vi "UHR-Fleezers Control (host) - 10.4.vi"() -> ()   [LabVIEW 2011] (continued)
                    n400 = Compound Arithmetic op=OR(w626, w627, w625) -> (w624:bool)
                    n401 = Select(t=FALSE, s=w623, f=w624) -> (s? t:f=w621:bool)
                    n402 = Not(x=w617) -> (.not. x?=w616:bool)
                    n403 = node-c288() -> ()  [unwired: 1 in, 1 out]
                    n404 = And(x=w620, y=w616) -> (x .and. y?=w618:bool)
                    n405 = Or(x=w621, y=w617) -> (x .or. y?=w619:bool)
                  }
                  n406 = node-c288(w611) -> ()  [unwired: 1 out]
                }
                frame #3 {
                  n407 = case shown="True" w636 {
                    tunnel: w635 -> [_ w638]
                    tunnel: w634 -> [_ w637]
                    frame False {
                    }
                    frame True {
                      n408 = flat-sequence {
                        tunnel: w638 -> [w641]
                        tunnel: w637 -> [w640]
                        frame #0 {
                          n409 = local read "Saved Stage Positions"() -> (w644:dbl[][])
                          n410 = local write "Cancel dwell"(FALSE ("Cancel dwell")) -> ()
                          n411 = call "move to saved stage position.vi"("error in"=w640, "Stage VISA resource name in"=w641, "Position"="Return Stage \nPosition", "Saved Stage Positions"=w644) -> ("error out"=w642:errorcluster)  [unwired: 1 out]
                          n412 = local write "Stage Control Serial Error"(w642) -> ()
                        }
                        frame #1 {
                          n413 = case shown="True" "Green ON \nafter return?" {
                            frame False {
                            }
                            frame True {
                              n414 = property on="Green Laser ON/Interlacing" class="Bool (strict)"("Val(Sgnl)"=TRUE ("Value (Signaling)")) -> ()  [unwired: 2 in, 2 out]
                            }
                          }
                          n415 = case shown="True" "Move trap \nafter return move?" {
                            frame False {
                            }
                            frame True {
                              n416 = property on="Trap Delta (MHz)" class="DigNum (strict)"("Val(Sgnl)"="Dip Trap Delta 2 (MHz)") -> ()  [unwired: 2 in, 2 out]
                            }
                          }
                          n417 = property on="Sample Channel\nFlow" class="Bool (strict)"("Val(Sgnl)"="Flow ON\nafter dip?") -> ()  [unwired: 2 in, 2 out]
                          n418 = case shown="True" "Save data\nafter return move?" {
                            frame False {
                            }
                            frame True {
                              n419 = property on="Start Saving" class="Bool (strict)"("Val(Sgnl)"=TRUE ("Value (Signaling)")) -> ()  [unwired: 2 in, 2 out]
                            }
                          }
                        }
                        frame #2 {
                          n420 = node-c288() -> (w653:T21)  [unwired: 4 in]
                          n421 = timed-loop {
                            timing: w653 -> [_]
                            timing-out: [_] -> w652
                            i -> [w665]
                            stop <- w655 stop-if-true
                            n422 = node-c288() -> ()  [unwired: 1 in, 1 out]
                            n423 = local read "Dump Beads"() -> (w654:bool)
                            n424 = Greater Or Equal?(x=w665, y="Dwell Duration (s)") -> (x >= y?=w660:bool)
                            n425 = local read "Dip for Protein"() -> (w657:bool)
                            n426 = Not(x=w657) -> (.not. x?=w656:bool)
                            n427 = Compound Arithmetic op=OR(w660, "Cancel dwell", w656) -> (w659:bool)
                            n428 = node-c288() -> ()  [unwired: 1 in, 1 out]
                            n429 = Select(t=FALSE, s="Pause dwell \ntimer", f=w659) -> (s? t:f=w662:bool)
                            n430 = Or(x=w662, y=w654) -> (x .or. y?=w655:bool)
                          }
                          n431 = node-c288(w652) -> ()  [unwired: 1 out]
                        }
                      }
                    }
                  }
                }
                frame #4 {
                  n432 = local read "Dip for Protein"() -> (w673:bool)
                  n433 = local read "Dump Beads"() -> (w670:bool)
                  n434 = local write "Cancel dwell"(FALSE ("Cancel dwell")) -> ()
                  n435 = Not(x=w673) -> (.not. x?=w674:bool)
                  n436 = Not(x="Cont. Repeat Dipping?") -> (.not. x?=w676:bool)
                  n437 = Compound Arithmetic op=OR(w674, w676, w670) -> (w672:bool)
                }
              }
            }
          }
        }
      }
      event "Profile": Value Change {
        n438 = event-data() -> ()  [unwired: 1 in, 5 out]
        n439 = flat-sequence {
          tunnel: w685 -> [w688]
          tunnel: w684 -> [w696]
          tunnel: [w690] -> w683
          tunnel: [w689] -> w682
          tunnel: [w687] -> w680
          tunnel: [w686] -> w677
          tunnel: w683 -> [w703]
          tunnel: w682 -> [w702]
          tunnel: [w700] -> w681
          tunnel: w680 -> [w701]
          tunnel: [w699] -> w679
          tunnel: [w698] -> w678
          tunnel: w677 -> [w698]
          tunnel: w681 -> [w707]
          tunnel: w679 -> [w706]
          tunnel: w678 -> [w705]
          frame #0 {
            n440 = call "Read Stage Position.vi"("error in"=w696, "VISA resource name in"=w688) -> ("Current Position"=w686:cluster{dbl, dbl, dbl}, "error out"=w689:errorcluster, "VISA resource name out"=w687:refnum<visa-resource-name>)  [unwired: 1 out]
            "Current Position" <- w686
            n441 = local write "Stage Control Serial Error"(w689) -> ()
            n442 = Unbundle(w686) -> (w693:dbl, w695:dbl, w691:dbl)
            n443 = Add(x=w695, y="Y change (mm)") -> (x+y=w692:dbl)
            n444 = Bundle(w693, w692, w691) -> (w690:cluster{dbl, dbl, dbl})  [unwired: 1 in]
          }
          frame #1 {
            # "move to new position and start saving"
            n445 = local write "Stage Moving"(TRUE ("Stage Moving")) -> ()
            n446 = local write "Start Saving"(TRUE ("Start Saving")) -> ()
            n447 = call "Set Stage Position.vi"("Position"=w703, "error in"=w702, "VISA resource name in"=w701) -> ("error out"=w699:errorcluster, "VISA resource name out"=w700:refnum<visa-resource-name>)  [unwired: 1 out]
          }
          frame #2 {
            # "go back to start"
            n448 = call "Set Stage Position.vi"("Position"=w705, "error in"=w706, "VISA resource name in"=w707) -> ()  [unwired: 3 out]
          }
          frame #3 {
            # "stop saving"
            n449 = local write "Stop Saving"(TRUE ("Stop Saving")) -> ()
            n450 = local write "Stage Moving"(FALSE ("Stage Moving")) -> ()
          }
        }
      }
      event "Move to Position 1", "Move to Position 2", "Move to Position 3", "Move to Position 4", "Move to Position 5", "Lower Ch. Cap.": Value Change {
        n451 = event-data() -> ()  [unwired: 1 in, 5 out]
        n452 = Or(x="Move to Position 5", y="Lower Ch. Cap.") -> (x .or. y?=w713:bool)
        n453 = Build Array("Move to Position 1", "Move to Position 2", "Move to Position 3", "Move to Position 4", w713) -> (w716:bool[])
        n454 = Boolean Array To Number(Boolean array=w716) -> (number=w715:u32)
        n455 = Logarithm Base 2(1:w715) -> (0:w714:dbl)
        n456 = flat-sequence {
          tunnel: w714 -> [w725]
          tunnel: w711 -> [w723]
          tunnel: w710 -> [w722]
          frame #0 {
            n457 = local read "Saved Stage Positions"() -> (w733:dbl[][])
            n458 = Array Subset(array=w733, index (row)=w725, length (row)=1 ("length"), index (col)=1 ("index"), length (col)=3 ("length")) -> (w730:dbl[][])
            n459 = Reshape Array(w730, 3 ("dimension size")) -> (w728:dbl[])
            n460 = Array To Cluster(array=w728) -> (cluster=w727:cluster{"[0]":dbl, "[1]":dbl, "[2]":dbl})
            n461 = call "Set Stage Position.vi"("Position"=w727, "error in"=w722, "VISA resource name in"=w723) -> ("error out"=w726:errorcluster)  [unwired: 2 out]
            n462 = local write "Stage Moving"(TRUE ("Stage Moving")) -> ()
            n463 = local write "Stage Control Serial Error"(w726) -> ()
          }
          frame #1 {
            n464 = local write "Stage Moving"(FALSE ("Stage Moving")) -> ()
            n465 = call <vilib>:"Beep.vi"() -> ()  [unwired: 3 in, 9 out]
          }
        }
      }
      event "Got ADig bead": Value Change {
        n466 = event-data() -> ()  [unwired: 1 in, 5 out]
        n467 = local read "Cap 1 Samp Flow ON"() -> (w736:bool)
        n468 = flat-sequence {
          tunnel: w736 -> [w738]
          frame #0 {
            n469 = case shown="True" w738 {
              frame False {
              }
              frame True {
                n470 = property on="Sample Channel\nFlow" class="Bool (strict)"("Val(Sgnl)"=TRUE ("Value (Signaling)")) -> ()  [unwired: 2 in, 2 out]
              }
            }
          }
          frame #1 {
            n471 = property on="Move Cap. 1 (DNA Bottom)" class="Bool (strict)"("Val(Sgnl)"=TRUE ("Value (Signaling)")) -> ()  [unwired: 2 in, 2 out]
            n472 = property on="Inject Pump 3" class="Bool (strict)"("Val(Sgnl)"=FALSE ("Value (Signaling)")) -> ()  [unwired: 2 in, 2 out]
          }
        }
      }
      event "Take Force FB Data\nScript": Value Change {
        n473 = event-data() -> ()  [unwired: 1 in, 5 out]
        n474 = flat-sequence {
          tunnel: w747 -> [w751]
          tunnel: w748 -> [w752]
          tunnel: [w752] -> w743
          tunnel: [w751] -> w742
          tunnel: w743 -> [w755]
          tunnel: w742 -> [w754]
          tunnel: ["Trap Trig Fl."] -> w744
          tunnel: [w780] -> w745
          tunnel: w744 -> [w780]
          tunnel: [w783] -> w746
          tunnel: w745 -> [w783]
          tunnel: w746 -> [w786]
          frame #0 {
            n475 = property on="Trap Delta (MHz)" class="DigNum (strict)"("Val(Sgnl)"="Trap Delta Before Moving") -> ()  [unwired: 2 in, 2 out]
          }
          frame #1 {
            n476 = local read "Saved Stage Positions"() -> (w757:dbl[][])
            n477 = local write "FB Trap Pos Offset"(0.0 ("FB Trap Pos Offset")) -> ()
            n478 = property on="Trap Pos. FB Offset Factor" class="DigNum (strict)"("Val(Sgnl)"=i64 0 ("Value (Signaling)")) -> ()  [unwired: 2 in, 2 out]
            n479 = local write "Stage Moving"(TRUE ("Stage Moving")) -> ()
            n480 = call "move to saved stage position.vi"("error in"=w754, "Stage VISA resource name in"=w755, "Position"="Stage Position To Establish FB", "Saved Stage Positions"=w757) -> ("error out"=w753:errorcluster)  [unwired: 1 out]
            n481 = local write "Stage Control Serial Error"(w753) -> ()
          }
          frame #2 {
            n482 = call <vilib>:"Beep.vi"() -> ()  [unwired: 3 in, 9 out]
            n483 = Multiply(x="Wait (s)", y=u32 1000 ("milliseconds to wait")) -> (x*y=w763:u32)
            n484 = property on="Trap Delta (MHz)" class="DigNum (strict)"("Val(Sgnl)"="Starting \nTrap Delta (MHz)") -> ()  [unwired: 2 in, 2 out]
            n485 = local write "Stage Moving"(FALSE ("Stage Moving")) -> ()
            n486 = Wait (ms)(milliseconds to wait=w763) -> ()  [unwired: 1 out]
            n487 = property on="Tab Control 2" class="TabCtl (strict)"("Val(Sgnl)"=T6."Feedback on Trap Position" ("Value (Signaling)")) -> ()  [unwired: 2 in, 2 out]
            n488 = property on="Tab Control" class="TabCtl (strict)"("Val(Sgnl)"=T4."Trap Control (RF)" ("Value (Signaling)")) -> ()  [unwired: 2 in, 2 out]
          }
          frame #3 {
            n489 = property on="Set Reading to\nSetpoint" class="Bool (strict)"("Val(Sgnl)"=TRUE ("Value (Signaling)")) -> ()  [unwired: 2 in, 2 out]
            n490 = Wait (ms)(milliseconds to wait=u32 500) -> ()  [unwired: 1 out]
          }
          frame #4 {
            n491 = property on="Trap Pos. FB ON" class="Bool (strict)"("Val(Sgnl)"=TRUE ("Value (Signaling)")) -> ()  [unwired: 2 in, 2 out]
            n492 = Wait (ms)(milliseconds to wait=u32 250) -> ()  [unwired: 1 out]
          }
          frame #5 {
            n493 = case shown="False" "Trap Trig Fl." {
              frame False {
                n494 = case shown="True" "Green ON after FB ON?" {
                  selector: "Green ON after FB ON?" -> [_ w779]
                  frame False {
                  }
                  frame True {
                    n495 = property on="Green Laser ON/Interlacing" class="Bool (strict)"("Val(Sgnl)"=w779) -> ()  [unwired: 2 in, 2 out]
                  }
                }
              }
              frame True {
              }
            }
            n496 = case shown="False" "Remove Action Offset" {
              tunnel: TRUE ("Value (Signaling)") -> [w776 w777]
              frame False {
                n497 = property on="Remove Unwinding Offset" class="Bool (strict)"("Val(Sgnl)"=w776) -> ()  [unwired: 2 in, 2 out]
              }
              frame True {
                n498 = property on="Remove Action Offset" class="Bool (strict)"("Val(Sgnl)"=w777) -> ()  [unwired: 2 in, 2 out]
              }
            }
            n499 = Wait (ms)(milliseconds to wait=u32 250) -> ()  [unwired: 1 out]
          }
          frame #6 {
            n500 = property on="Start Saving" class="Bool (strict)"("Val(Sgnl)"=TRUE ("Value (Signaling)")) -> ()  [unwired: 2 in, 2 out]
            n501 = Wait (ms)(milliseconds to wait=u32 5000) -> ()  [unwired: 1 out]
          }
          frame #7 {
            n502 = property on="Rem fb disp offset" class="Bool (strict)"("Val(Sgnl)"=TRUE ("Value (Signaling)")) -> ()  [unwired: 2 in, 2 out]
            n503 = Wait (ms)(milliseconds to wait=u32 100) -> ()  [unwired: 1 out]
          }
          frame #8 {
            n504 = case shown="True" w786 {
              frame False {
              }
              frame True {
                n505 = local write "Trap Trig. Fl."(TRUE ("Value (Signaling)")) -> ()
              }
            }
          }
          frame #9 {
            n506 = case shown="True" "Start dipping after?" {
              frame False {
              }
              frame True {
                n507 = property on="Dip for Protein" class="Bool (strict)"("Val(Sgnl)"=TRUE ("Value (Signaling)")) -> ()  [unwired: 2 in, 2 out]
                n508 = local write "Scripts"(T1."Dipping" ("Scripts")) -> ()
              }
            }
          }
        }
      }
      event "Test move stage": Value Change {
        n509 = event-data() -> ()  [unwired: 1 in, 5 out]
        n510 = local read "Saved Stage Positions"() -> (w791:dbl[][])
        n511 = call "move to saved stage position.vi"("error in"=w792, "Stage VISA resource name in"=w793, "Saved Stage Positions"=w791) -> ()  [unwired: 1 in, 2 out]
      }
      event "Got DNA bead": Value Change {
        n512 = event-data() -> ()  [unwired: 1 in, 5 out]
        n513 = flat-sequence {
          frame #0 {
            n514 = local read "Daq spot flow on"() -> (w796:bool)
            n515 = case shown="True" w796 {
              frame False {
              }
              frame True {
                n516 = property on="Sample Channel\nFlow" class="Bool (strict)"("Val(Sgnl)"=TRUE ("Value (Signaling)")) -> ()  [unwired: 2 in, 2 out]
              }
            }
          }
          frame #1 {
            n517 = property on="Cal/Data Acq. Spot" class="Bool (strict)"("Val(Sgnl)"=TRUE ("Value (Signaling)")) -> ()  [unwired: 2 in, 2 out]
            n518 = property on="Inject Pump 1" class="Bool (strict)"("Val(Sgnl)"=FALSE ("Value (Signaling)")) -> ()  [unwired: 2 in, 2 out]
          }
        }
      }
      event "Take Stepping Data": Value Change {
        n519 = event-data() -> ()  [unwired: 1 in, 5 out]
        n520 = local read "Save ave N"() -> (w808:dbl)
        n521 = flat-sequence {
          tunnel: w808 -> [w810]
          tunnel: [w810] -> w803
          tunnel: [w812] -> w804
          tunnel: w803 -> [w812]
          tunnel: [w814] -> w805
          tunnel: w804 -> [w814]
          tunnel: [w817] -> w806
          tunnel: w805 -> [w817]
          tunnel: [w819] -> w807
          tunnel: w806 -> [w819]
          tunnel: [w821] -> w801
          tunnel: w807 -> [w821]
          tunnel: w801 -> [w824]
          tunnel: [w824] -> w800
          tunnel: w800 -> [w825]
          tunnel: [w825] -> w802
          tunnel: w802 -> [w831]
          frame #0 {
            n522 = property on="Save ave N" class="DigNum (strict)"("Val(Sgnl)"="Save ave factor") -> ()  [unwired: 2 in, 2 out]
          }
          frame #1 {
            n523 = Wait (ms)(milliseconds to wait=u32 100) -> ()  [unwired: 1 out]
          }
          frame #2 {
            n524 = local read "Offset 2 Start (MHz)"() -> (w816:dbl)
            n525 = property on="Saved AOD Raster Scan Parameter Sets" class="Arr (strict)"("Index Values"=u32[] [2]) -> ()  [unwired: 2 in, 2 out]
            n526 = property on="Trap Delta (MHz)" class="DigNum (strict)"("Val(Sgnl)"=w816) -> ()  [unwired: 2 in, 2 out]
          }
          frame #3 {
            n527 = property on="Load parameters" class="Bool (strict)"("Val(Sgnl)"=TRUE ("Value (Signaling)")) -> ()  [unwired: 2 in, 2 out]
          }
          frame #4 {
            n528 = Wait (ms)(milliseconds to wait=u32 100) -> ()  [unwired: 1 out]
          }
          frame #5 {
            n529 = property on="Trap Raster Scan" class="Bool (strict)"("Val(Sgnl)"=TRUE ("Value (Signaling)")) -> ()  [unwired: 2 in, 2 out]
          }
          frame #6 {
            n530 = Wait (ms)(milliseconds to wait=u32 1000) -> ()  [unwired: 1 out]
          }
          frame #7 {
            n531 = while {
              stop <- w828 stop-if-true
              n532 = local read "Raster Scanning..."() -> (w830:bool)
              n533 = local read "Saving..."() -> (w829:bool)
              n534 = Not(x=w829) -> (.not. x?=w826:bool)
              n535 = Not(x=w830) -> (.not. x?=w827:bool)
              n536 = And(x=w827, y=w826) -> (x .and. y?=w828:bool)
            }
          }
          frame #8 {
            n537 = property on="Save ave N" class="DigNum (strict)"("Val(Sgnl)"=w831) -> ()  [unwired: 2 in, 2 out]
          }
        }
      }
      event "Step Size (nm)": Value Change {
        n538 = event-data() -> ()  [unwired: 1 in, 5 out]
        n539 = flat-sequence {
          frame #0 {
            n540 = property on="Saved AOD Raster Scan Parameter Sets" class="Arr (strict)"("Index Values"=u32[] [1]) -> ()  [unwired: 2 in, 2 out]
          }
          frame #1 {
            n541 = Multiply(x="N Steps", y="Step Size (nm)") -> (x*y=w833:dbl)
            n542 = property on="Scan Speed AOD (nm/s) 2" class="DigNum (strict)"("Value"="Step Size (nm)") -> ()  [unwired: 2 in, 2 out]
            n543 = property on="Step Size AOD (nm) 2" class="DigNum (strict)"("Value"="Step Size (nm)") -> ()  [unwired: 2 in, 2 out]
            n544 = property on="Scan Range AOD (nm) 2" class="DigNum (strict)"("Value"=w833) -> ()  [unwired: 2 in, 2 out]
          }
        }
      }
      event "Take Detection Laser\nImage": Value Change {
        n545 = event-data() -> ()  [unwired: 1 in, 5 out]
        n546 = flat-sequence {
          tunnel: [w861] -> w851
          tunnel: [w860] -> w844
          tunnel: [w859] -> w836
          tunnel: [w864] -> w852
          tunnel: w851 -> [w864]
          tunnel: [w863] -> w845
          tunnel: w844 -> [w863]
          tunnel: [w862] -> w837
          tunnel: w836 -> [w862]
          tunnel: [w868] -> w853
          tunnel: w852 -> [w868]
          tunnel: [w867] -> w846
          tunnel: w845 -> [w867]
          tunnel: [w866] -> w838
          tunnel: w837 -> [w866]
          tunnel: [w874] -> w854
          tunnel: w853 -> [w874]
          tunnel: [w873] -> w847
          tunnel: w846 -> [w873]
          tunnel: [w872] -> w839
          tunnel: w838 -> [w872]
          tunnel: [w878] -> w855
          tunnel: w854 -> [w878]
          tunnel: [w877] -> w848
          tunnel: w847 -> [w877]
          tunnel: [w876] -> w840
          tunnel: w839 -> [w876]
          tunnel: [w882] -> w856
          tunnel: w855 -> [w882]
          tunnel: [w881] -> w849
          tunnel: w848 -> [w881]
          tunnel: [w880] -> w841
          tunnel: w840 -> [w880]
          tunnel: [w886] -> w857
          tunnel: w856 -> [w886]
          tunnel: [w885] -> w850
          tunnel: w849 -> [w885]
          tunnel: [w884] -> w842
          tunnel: w841 -> [w884]
          tunnel: w857 -> [w892]
          tunnel: w850 -> [w891]
          tunnel: [w889] -> w843
          tunnel: w842 -> [w889]
          tunnel: w843 -> [w893]
          frame #0 {
            n547 = local read "Green Laser ON/Interlacing"() -> (w861:bool)
            n548 = local read "Green laser mode"() -> (w860:enum32{"Laser ON", "Laser OFF", "Interlace"})
            n549 = local read "Green FB On/Off"() -> (w859:bool)
          }
          frame #1 {
            n550 = property on="Green FB On/Off" class="Bool (strict)"("Val(Sgnl)"=FALSE ("Value (Signaling)")) -> ()  [unwired: 2 in, 2 out]
          }
          frame #2 {
            n551 = property on="Green Laser ON/Interlacing" class="Bool (strict)"("Val(Sgnl)"=TRUE ("Value (Signaling)")) -> ()  [unwired: 2 in, 2 out]
            n552 = property on="Flip Green Filter" class="Bool (strict)"("Val(Sgnl)"=TRUE ("Value (Signaling)")) -> ()  [unwired: 2 in, 2 out]
            n553 = property on="Green laser mode" class="RadioBtnsControl (strict)"("Val(Sgnl)"=enum32{"Laser ON", "Laser OFF", "Interlace"}."Laser ON" ("Value (Signaling)")) -> ()  [unwired: 2 in, 2 out]
          }
          frame #3 {
            n554 = Wait (ms)(milliseconds to wait=u32 500) -> ()  [unwired: 1 out]
          }
          frame #4 {
            n555 = property on="Confocal Image" class="Bool (strict)"("Val(Sgnl)"=TRUE ("Value (Signaling)")) -> ()  [unwired: 2 in, 2 out]
          }
          frame #5 {
            n556 = Wait (ms)(milliseconds to wait=u32 2000) -> ()  [unwired: 1 out]
          }
          frame #6 {
            n557 = while {
              stop <- w887 stop-if-true
              n558 = local read "Saving..."() -> (w888:bool)
              n559 = Not(x=w888) -> (.not. x?=w887:bool)
            }
          }
          frame #7 {
            n560 = property on="Flip Green Filter" class="Bool (strict)"("Val(Sgnl)"=TRUE ("Value (Signaling)")) -> ()  [unwired: 2 in, 2 out]
            n561 = property on="Green Laser ON/Interlacing" class="Bool (strict)"("Val(Sgnl)"=w892) -> ()  [unwired: 2 in, 2 out]
            n562 = property on="Green laser mode" class="RadioBtnsControl (strict)"("Val(Sgnl)"=w891) -> ()  [unwired: 2 in, 2 out]
          }
          frame #8 {
            n563 = property on="Green FB On/Off" class="Bool (strict)"("Val(Sgnl)"=w893) -> ()  [unwired: 2 in, 2 out]
          }
        }
      }
      event "Stop All": Value Change {
        n564 = event-data() -> ()  [unwired: 1 in, 5 out]
        n565 = local read "Stop All"() -> (w894:bool)
      }
    }
    n566 = node-c288() -> ()  [unwired: 1 in, 1 out]
  }
  n567 = node-c288(2 ("Processor")) -> (w80:T21)  [unwired: 3 out]
  n568 = timed-loop "Control parameters (event loop)" {
    tunnel: w38 -> [w899]
    shift-right: [w898] -> _
    shift-left: errorcluster {"status"=FALSE, "code"=0, "source"=""} ("error out") -> [w897]
    tunnel: [w896] -> _
    timing: w80 -> [_]
    timing-out: [_] -> w79
    tunnel: w52 -> [w895]
    stop <- w896 stop-if-true
    n569 = node-c288() -> ()  [unwired: 2 out]
    n570 = event shown="[54] \"11\": Value Change" {
      selector: _ -> [_ _ _ _ _ _ _ _ _ _ _ _ _ _ _ _ _ _ _ _ _ _ _ _ _ _ _ _ _ _ _ _ _ _ _ _ _ _ _ _ _ _ _ _ _ _ _ _ _ _ _ _ _ _ _ _ _ _ _ _ _ _ _]
      dyn-events: _ -> [_ _ _ _ _ _ _ _ _ _ _ _ _ _ _ _ _ _ _ _ _ _ _ _ _ _ _ _ _ _ _ _ _ _ _ _ _ _ _ _ _ _ _ _ _ _ _ _ _ _ _ _ _ _ _ _ _ _ _ _ _ _ _]
      timeout: _ -> [_ _ _ _ _ _ _ _ _ _ _ _ _ _ _ _ _ _ _ _ _ _ _ _ _ _ _ _ _ _ _ _ _ _ _ _ _ _ _ _ _ _ _ _ _ _ _ _ _ _ _ _ _ _ _ _ _ _ _ _ _ _ _]
      tunnel: w899 -> [w937 _ _ _ w974 _ w996 _ _ _ _ w1062 _ _ w1105 w1111 w1116 w1122 w1158 w1176 w1183 w1194 w1198 w1209 w1220 w1231 w1242 w1253 w1264 w1291 w1385 w1392 w1430 _ w1465 w1469 w1480 w1484 w1488 _ w1496 _ _ _ _ _ _ _ w1667 _ w1684 _ w1691 w1709 _ w1716 w1724 w1739 w1748 w1751 w1756 _ w1772]
      tunnel: [w936 _ _ _ w964 _ w995 _ _ w1027 _ w1041 _ _ w1104 w1107 w1113 w1119 w1157 w1174 w1182 w1192 _ w1203 w1214 w1225 w1236 w1247 w1258 w1289 w1383 w1390 w1428 _ w1463 w1467 w1470 w1482 w1486 _ w1494 _ _ _ _ _ _ _ w1665 _ _ _ _ w1706 _ _ _ _ _ _ _ _ _] -> w898
      tunnel: w897 -> [w935 _ _ _ w973 _ w994 _ _ w1027 _ w1061 _ _ w1103 w1106 w1112 w1118 w1156 w1175 w1181 w1193 w1197 w1208 w1219 w1230 w1241 w1252 w1263 w1290 w1384 w1391 w1429 _ w1464 w1468 w1479 w1483 w1487 _ w1495 _ _ _ _ _ _ _ w1666 _ w1683 _ w1690 w1708 _ w1715 w1723 w1738 w1747 w1750 w1755 _ w1771]
      tunnel: [_ _ _ _ _ _ _ _ _ w1026 _ _ _ _ _ _ _ _ _ _ _ _ _ _ _ _ _ _ _ _ _ _ _ _ _ _ _ _ _ _ _ _ _ _ _ _ _ _ _ _ _ _ _ _ _ _ _ _ _ _ _ _ _] -> w896
      tunnel: [_ _ _ _ _ _ _ "Round T1 X" _ _ _ _ _ _ _ _ _ _ _ _ _ _ _ _ _ _ _ _ _ _ _ _ _ _ _ _ _ _ _ _ _ _ _ _ _ _ _ _ _ _ _ _ _ _ _ _ _ _ _ _ _ _ _] -> _
      tunnel: [_ _ _ "Adjust Scale\nto Mean" _ _ _ _ _ _ _ _ _ _ _ _ _ _ _ _ _ "Test ttrig" _ _ _ _ _ _ _ _ _ _ _ _ _ _ _ _ _ _ _ _ _ _ _ _ "Flush Sample" "Clear Volume" _ _ _ _ _ _ _ _ _ _ _ _ _ _ _] -> _
      tunnel: [_ _ _ _ _ _ _ _ "Round T2 X" _ "Delayed Interlace Start" _ _ _ _ _ _ _ _ _ _ _ _ _ _ _ _ _ _ _ _ _ _ _ _ _ _ _ _ _ _ _ _ _ _ _ _ _ _ _ _ _ _ _ _ _ _ _ _ _ _ _ _] -> _
      tunnel: w895 -> [_ _ _ _ _ _ _ _ _ _ _ _ _ _ _ _ _ _ _ _ _ _ _ _ _ _ _ _ _ _ _ _ _ _ _ _ _ _ _ _ _ _ _ _ w1609 w1624 w1652 w1654 _ _ _ _ _ _ _ _ _ _ _ _ _ _ _]
      event "AI Count (ticks)", "Sets to FIFO (Traps)", "Save ave N", "FPGA Ave.", "# Samples/channel", "N sets to save": Value Change {
        # "So that if 'Save ave N' is updated, the AOD scanning code updates too."
        n571 = event-data() -> ()  [unwired: 6 out]
        n572 = local read "AI Count (ticks)"() -> (w917:u32)
        n573 = Boolean To (0,1)(Boolean="Sets to FIFO (Traps)") -> (0, 1=w927:cluster{"Set 1":i16, "Set 2":i16, "Set 3":i16})
        n574 = xnode "Read/Write Control"("FPGA VI Reference In"=w937, "error in"=w935, "ai count"=w917, "AI1 Sets to FIFO"="Sets to FIFO (Traps)", "N of AI1 Int Acq Sets"="N Acq Sets (Traps + Fl.)") -> ("error out"=w936:errorcluster)  [unwired: 1 out]
        n575 = Cluster To Array(cluster=w927) -> (array=w926:i16[])
        n576 = To Unsigned Long Integer(number=w926) -> (unsigned 32bit integer=w906:u32[])
        n577 = local read "Scan steps (AOD)"() -> (w928:u64)
        n578 = Multiply(x=w917, y="N Acq Sets (Traps + Fl.)") -> (x*y=w915:u32)
        n579 = Divide(x=40000000.0, y=w917) -> (x/y=w909:dbl)
        "AI rate (Hz)" <- w909
        "Ave. Rate (Hz)" <- w909
        n580 = Add Array Elements(numeric array=w906) -> (sum=w918:u32)
        "Trap Sets" <- w918
        n581 = Reciprocal(x=w909) -> (1/x=→"Ave. Period (s)":dbl)
        n582 = property on="Scan steps (AOD)" class="DigNum (strict)"("Val(Sgnl)"=w928) -> ()  [unwired: 2 in, 2 out]
        n583 = Divide(x=w909, y="N Acq Sets (Traps + Fl.)") -> (x/y=w932:dbl)
        "Data Rate (Hz)" <- w932
        n584 = Reciprocal(x=w932) -> (1/x=→"Data Period (s)":dbl)
        n585 = local read "Save ave N"() -> (w931:dbl)
        n586 = Divide(x=w932, y=w931) -> (x/y=w930:dbl)
        "Save Data Rate (Hz)" <- w930
        n587 = Reciprocal(x=w930) -> (1/x=→"Save Data Period (s)":dbl)
        n588 = Multiply(x=w915, y="# Samples/trap") -> (x*y=w913:u32)
        "Counts/DMA" <- w913
        n589 = property on="Trap Disp. Downsample" class="DigNum (strict)"("Maximum"="# Samples/trap") -> ()  [unwired: 2 in, 2 out]
        n590 = Multiply(x=w918, y="# Samples/trap") -> (x*y=w907:u32)
        "# Samples/channel" <- w907
        n591 = Multiply(x=w907, y=u32 8) -> (x*y=→"Trap AI Elements/DMA read":u32)
        n592 = local read "APD Int. Count"() -> (w914:u32)
        n593 = Multiply(x=w907, y=u32 3) -> (x*y=→"Trap Pos Elements/DMA read":u32)
        n594 = Divide(x=w913, y=w914) -> (x/y=w904:dbl)
        "APD Samples/FIFO Acq." <- w904
        n595 = Divide(x=w913, y=40000000.0) -> (x/y=w911:dbl)
        "DMA Update Period (s)" <- w911
        n596 = Multiply(x=2.0, y=w904) -> (x*y=→"APD Elements/DMA read":dbl)
        n597 = property on="APD Disp. Downsample" class="DigNum (strict)"("Maximum"=w904) -> ()  [unwired: 2 in, 2 out]
        n598 = local read "N sets to save"() -> (w924:u32)
        n599 = Multiply(x=w911, y=w924) -> (x*y=→"Total Time (s)":dbl)
        "FPGA Averaging" <- FALSE ("FPGA Averaging")
      }
      event "Rescale on Mean": Value Change {
        n600 = event-data() -> ()  [unwired: 7 out]
        n601 = And(x=FALSE, y="Rescale on Mean") -> (x .and. y?=w939:bool)
        n602 = local write "Rescale on Mean"(w939) -> ()
        n603 = local read "Bead Mean (nm)"() -> (w944:dbl)
        n604 = Add(x="Amplitude (nm)", y=w944) -> (x+y=w942:dbl)
        n605 = Subtract(x=w944, y="Amplitude (nm)") -> (x-y=w941:dbl)
        n606 = property on="Bead Separation" class="WFChart (strict)"("YScale.Minimum"=w941) -> ()  [unwired: 2 in, 2 out]
        n607 = property on="Bead Separation" class="WFChart (strict)"("YScale.Maximum"=w942) -> ()  [unwired: 2 in, 2 out]
      }
      event "Detector Type": Value Change {
        n608 = event-data() -> ()  [unwired: 7 out]
        n609 = local read "AI labels"() -> (w945:string[])
        n610 = property on="High Res. Display" class="Ring (strict)"("Strings []"=w945) -> ()  [unwired: 2 in, 2 out]
        n611 = Build Array (concatenate)(w945, "none") -> (w946:string[])
        n612 = property on="FFT 1 Choice 1" class="Ring (strict)"("Strings []"=w946) -> ()  [unwired: 2 in, 2 out]
        n613 = property on="FFT 1 Choice 2" class="Ring (strict)"("Strings []"=w946) -> ()  [unwired: 2 in, 2 out]
        n614 = property on="FFT 2 Choice 1" class="Ring (strict)"("Strings []"=w946) -> ()  [unwired: 2 in, 2 out]
        n615 = property on="FFT 2 Choice 2" class="Ring (strict)"("Strings []"=w946) -> ()  [unwired: 2 in, 2 out]
        n616 = Bundle("APD 1", "APD 2") -> (w949:cluster{string, string})  [unwired: 1 out]
        n617 = Cluster To Array(cluster=w949) -> (array=w947:string[])
        n618 = Build Array (concatenate)(w947, w946) -> (w951:string[])
        n619 = Array Size(array=w951) -> (size(s)=w952:i32)
        n620 = property on="Signals to Plot" class="LstBox (strict)"("Item Names"=w951) -> ()  [unwired: 2 in, 2 out]
        n621 = property on="Signals to Plot" class="LstBox (strict)"("Number of Rows"=w952) -> ()  [unwired: 2 in, 2 out]
        n622 = property on="All Signals" class="WFChart (strict)"("LegNumRows"=w952) -> ()  [unwired: 2 in, 2 out]
      }
      event "Adjust Scale\nto Mean": Value Change {
        n623 = event-data() -> ()  [unwired: 7 out]
        n624 = local read "APD 1 Rate (Hz)"() -> (w961:dbl)
        n625 = Multiply(x=1000.0, y="Above (kHz)") -> (x*y=w959:dbl)
        n626 = Multiply(x=1000.0, y="Below (kHz)") -> (x*y=w957:dbl)
        n627 = Add(x=w959, y=w961) -> (x+y=w954:dbl)
        n628 = Subtract(x=w961, y=w957) -> (x-y=w955:dbl)
        n629 = property on="APD Chart" class="WFChart (strict)"("YScale.Minimum"=w955) -> ()  [unwired: 2 in, 2 out]
        n630 = property on="APD Chart" class="WFChart (strict)"("YScale.Maximum"=w954) -> ()  [unwired: 2 in, 2 out]
      }
      event "Phase adj. (AI1)", "+ phase (AI1)", "- phase (AI1)": Value Change {
        n631 = event-data() -> ()  [unwired: 7 out]
        n632 = Negate(x="Phase adj. (AI1)") -> (-x=w971:i16)
        n633 = Select(t=w971, s="- phase (AI1)", f="Phase adj. (AI1)") -> (s? t:f=w970:i16)
        n634 = xnode "Read/Write Control"("FPGA VI Reference In"=w974, "error in"=w973, "Phase count adjustment"=w970) -> ("FPGA VI Reference Out"=w969:T19, "error out"=w968:errorcluster)
        n635 = Or(x="- phase (AI1)", y="+ phase (AI1)") -> (x .or. y?=w965:bool)
        n636 = xnode "Read/Write Control"("FPGA VI Reference In"=w969, "error in"=w968, "+ phase"=w965) -> ("error out"=w964:errorcluster)  [unwired: 1 out]
      }
      event "Signals to Plot": Double Click {
        w977 = u32 9868950 ("Color Box")
        n637 = event-data() -> ("Row"=w979:i32)  [unwired: 9 out]
        n638 = property on="All Signals" class="WFChart (strict)"("Active Plot"=w979) -> (error out=w990:errorcluster)  [unwired: 2 in, 1 out]
        n639 = property on="All Signals" class="WFChart (strict)" props=["Plot", "Visible?", "Plot", "Plot Color"](error in=w990) -> (error out=w989:errorcluster, "Plot.Visible?"=w988:bool)  [unwired: 1 in, 2 out]
        n640 = Select(t=FALSE ("Plot.Visible"), s=w988, f=TRUE ("Plot.Visible")) -> (s? t:f=w983:bool)
        n641 = property on="All Signals" class="WFChart (strict)"(error in=w989, "Plot.Visible?"=w983) -> (error out=w985:errorcluster)  [unwired: 1 in, 1 out]
        n642 = property on="All Signals" class="WFChart (strict)"(error in=w985) -> (error out=w980:errorcluster, "Plot.Plot Color"=w984:u32)  [unwired: 1 in, 1 out]
        n643 = property on="Signals to Plot" class="LstBox (strict)"(error in=w980, "Active Row"=w979) -> (error out=w978:errorcluster)  [unwired: 1 in, 1 out]
        n644 = Select(t=w984, s=w983, f=u32 0) -> (s? t:f=w981:u32)
        n645 = property on="Signals to Plot" class="LstBox (strict)"(error in=w978, "CellFontColor"=w981, "SelColor"=w977, "CellBG"=w977, "CellFontSize"=u32 20 ("Active Row:Cell Font:Size"), "CellFontBold"=TRUE ("Active Row:Cell Font:Bold")) -> ()  [unwired: 1 in, 2 out]
      }
      event "BD 1 Frequency 1 (MHz)", "BD 1 Frequency 2 (MHz)", "BD 1 Frequency 3 (MHz)", "BD 2 Frequency 1 (MHz)", "BD 2 Frequency 2 (MHz)", "BD 2 Frequency 3 (MHz)", "Trap Delta (MHz)": Value Change {
        n646 = event-data() -> ("CtlRef"=w993:refnum<vi>)  [unwired: 6 out]
        n647 = control-ref of="Trap Delta (MHz)"() -> (w992:refnum<vi>)
        n648 = Equal?(x=w992, y=w993) -> (x = y?=w991:bool)
        n649 = case shown="False" "Oscillate Set 1" {
          tunnel: w996 -> [w1016 _]
          tunnel: [w1015 w1019] -> w995
          tunnel: w994 -> [w1014 w1019]
          tunnel: w991 -> [w999 _]
          frame False {
            n650 = local read "BD 1 Frequency 2 (MHz)"() -> (w1003:dbl)
            n651 = local read "BD 1 Frequency 1 (MHz)"() -> (w1001:dbl)
            n652 = Subtract(x=w1003, y="Trap Delta (MHz)") -> (x-y=w1000:dbl)
            n653 = Select(t=w1000, s=w999, f=w1001) -> (s? t:f=w998:dbl)
            n654 = local read "Y RF Frequency Limits (MHz)"() -> (w1004:T16)
            n655 = local read "X RF Frequency Limits (MHz)"() -> (w1005:T16)
            n656 = local read "BD 1 Frequency 3 (MHz)"() -> (w1017:dbl)
            n657 = local write "BD 1 Frequency 1 (MHz)"(w998) -> ()
            n658 = local read "BD 2 Frequency 1 (MHz)"() -> (w1008:dbl)
            n659 = local read "BD 2 Frequency 2 (MHz)"() -> (w1007:dbl)
            n660 = local read "BD 2 Frequency 3 (MHz)"() -> (w1018:dbl)
            n661 = call "set RF board frequency - interlace.vi"("Board 2 Frequency Limits"=w1004, "Board 1 Frequency Limits"=w1005, "error in"=w1014, "FPGA VI Reference In"=w1016, "Board 2 Frequency 3 (MHz)"=w1018, "Board 1 Frequency 3 (MHz)"=w1017, "Board 2 Frequency 2 (MHz)"=w1007, "Board 2 Frequency 1 (MHz)"=w1008, "Board 1 Frequency 2 (MHz)"=w1003, "Board 1 Frequency 1  (MHz)"=w998) -> ("error out"=w1015:errorcluster)  [unwired: 1 out]
            n662 = Subtract(x=w1008, y=w1007) -> (x-y=w1012:dbl)
            n663 = Subtract(x=w998, y=w1003) -> (x-y=w1013:dbl)
            n664 = Square(x=w1012) -> (x^2=w1010:dbl)
            n665 = Square(x=w1013) -> (x^2=w1011:dbl)
            n666 = Add(x=w1011, y=w1010) -> (x+y=w1009:dbl)
            n667 = Square Root(x=w1009) -> (sqrt(x)=w1006:dbl)
            n668 = local write "Trap Delta (MHz)"(w1006) -> ()
            n669 = property on="Initial delta (MHz)" class="DigNum (strict)"("Val(Sgnl)"=w1006) -> ()  [unwired: 2 in, 2 out]
          }
          frame True {
          }
        }
      }
      event "Round T1 X": Value Change {
        n670 = event-data() -> ()  [unwired: 7 out]
        n671 = local read "BD 1 Frequency 1 (MHz)"() -> (w1022:dbl)
        n672 = Round To Nearest(number=w1022) -> (nearest integer value=w1021:dbl)
        n673 = property on="BD 1 Frequency 1 (MHz)" class="DigNum (strict)"("Val(Sgnl)"=w1021) -> ()  [unwired: 2 in, 2 out]
      }
      event "Round T2 X": Value Change {
        n674 = event-data() -> ()  [unwired: 7 out]
        n675 = local read "BD 1 Frequency 2 (MHz)"() -> (w1024:dbl)
        n676 = Round To Nearest(number=w1024) -> (nearest integer value=w1023:dbl)
        n677 = property on="BD 1 Frequency 2 (MHz)" class="DigNum (strict)"("Val(Sgnl)"=w1023) -> ()  [unwired: 2 in, 2 out]
      }
      event "Stop All": Value Change {
        n678 = event-data() -> ()  [unwired: 7 out]
        n679 = local read "Stop All"() -> (w1026:bool)
      }
      event "Delayed Interlace Start": Value Change {
        n680 = event-data() -> ()  [unwired: 7 out]
        n681 = flat-sequence {
          frame #0 {
            n682 = Multiply(x="Delay to Interlace (s)", y=1000.0) -> (x*y=w1029:dbl)
            n683 = Wait (ms)(milliseconds to wait=w1029) -> ()  [unwired: 1 out]
          }
          frame #1 {
            n684 = property on="Green laser mode" class="RadioBtnsControl (strict)"("Val(Sgnl)"=enum32{"Laser ON", "Laser OFF", "Interlace"}."Interlace" ("Value (Signaling)")) -> ()  [unwired: 2 in, 2 out]
          }
        }
      }
      event "BD 1 Amplitude 1 (%)", "BD 1 Amplitude 2 (%)", "BD 1 Amplitude 3 (%)", "BD 2 Amplitude 1 (%)", "BD 2 Amplitude 2 (%)", "BD 2 Amplitude 3 (%)", "Trap 1 ON", "Trap 2 ON", "Trap 3 ON", "Feedback On/Off", "All FB On/Off": Value Change {
        w1053 = i16 1 ("f")
        n685 = event-data() -> ()  [unwired: 7 out]
        n686 = local write "Trap 1 (ON/OFF)"("Trap 1 ON") -> ()
        n687 = local write "Trap 2 (ON/OFF)"("Trap 2 ON") -> ()
        n688 = Boolean To (0,1)(Boolean="Trap 3 ON") -> (0, 1=w1054:i16)
        n689 = Boolean To (0,1)(Boolean="Trap 1 ON") -> (0, 1=w1055:i16)
        n690 = Boolean To (0,1)(Boolean="Trap 2 ON") -> (0, 1=w1056:i16)
        n691 = Select(t=w1056, s="Trap ON/OFF X or Y Amp?", f=w1053) -> (s? t:f=w1051:i16)
        n692 = Select(t=w1055, s="Trap ON/OFF X or Y Amp?", f=w1053) -> (s? t:f=w1052:i16)
        n693 = Select(t=w1054, s="Trap ON/OFF X or Y Amp?", f=w1053) -> (s? t:f=w1050:i16)
        n694 = Select(t=w1053, s="Trap ON/OFF X or Y Amp?", f=w1056) -> (s? t:f=w1048:i16)
        n695 = Select(t=w1053, s="Trap ON/OFF X or Y Amp?", f=w1055) -> (s? t:f=w1049:i16)
        n696 = Select(t=w1053, s="Trap ON/OFF X or Y Amp?", f=w1054) -> (s? t:f=w1047:i16)
        n697 = And(x="All FB On/Off", y="Feedback On/Off") -> (x .and. y?=w1045:cluster{"Set 1":bool, "Set 2":bool})
        n698 = local read "BD 1 Amplitude 1 (%)"() -> (w1065:dbl)
        n699 = local read "BD 1 Amplitude 2 (%)"() -> (w1064:dbl)
        n700 = local read "BD 1 Amplitude 3 (%)"() -> (w1063:dbl)
        n701 = Unbundle By Name(w1045) -> ("Set 1"=w1040:bool, "Set 2"=w1037:bool)
        n702 = local read "Y RF Amplitude Limits (%)"() -> (w1033:T16)
        n703 = local read "X RF Amplitude Limits (%)"() -> (w1034:T16)
        n704 = local read "BD 2 Amplitude 1 (%)"() -> (w1066:dbl)
        n705 = local read "BD 2 Amplitude 2 (%)"() -> (w1067:dbl)
        n706 = local read "BD 2 Amplitude 3 (%)"() -> (w1068:dbl)
        n707 = And(x="Trap 2 ON", y=w1037) -> (x .and. y?=w1035:bool)
        n708 = And(x="Trap 1 ON", y=w1040) -> (x .and. y?=w1038:bool)
        n709 = Multiply(x=w1052, y=w1065) -> (x*y=w1060:dbl)
        n710 = Multiply(x=w1064, y=w1051) -> (x*y=w1058:dbl)
        n711 = Multiply(x=w1063, y=w1050) -> (x*y=w1059:dbl)
        n712 = Multiply(x=w1066, y=w1049) -> (x*y=w1069:dbl)
        n713 = Multiply(x=w1067, y=w1048) -> (x*y=w1070:dbl)
        n714 = Multiply(x=w1068, y=w1047) -> (x*y=w1071:dbl)
        n715 = call "set RF board amplitude - interlace.vi"("Board 2 Amplitude Limits"=w1033, "Board 1 Amplitude Limits"=w1034, "error in"=w1061, "FPGA VI Reference In"=w1062, "Board 2 Amplitude 3 (%)"=w1071, "Board 1 Amplitude 3 (%)"=w1059, "Board 2 Amplitude 2 (%)"=w1070, "Board 2 Amplitude 1 (%)"=w1069, "Board 1 Amplitude 2 (%)"=w1058, "Board 1 Amplitude 1 (%)"=w1060) -> ("error out"=w1042:errorcluster, "FPGA VI Reference Out"=w1043:T19)
        n716 = xnode "Read/Write Control"("FPGA VI Reference In"=w1043, "error in"=w1042, "FB On/Off Set 1"=w1038, "FB On/Off Set 2"=w1035) -> ("error out"=w1041:errorcluster)  [unwired: 1 out]
      }
      event "Load parameters": Value Change {
        n717 = event-data() -> ()  [unwired: 7 out]
        n718 = property on="Saved AOD Raster Scan Parameter Sets" class="Arr (strict)"() -> ("Index Values"=w1082:u32[])  [unwired: 2 in, 2 out]
        n719 = Index Array(array=w1082, index=0) -> (element=w1079:u32)
        n720 = local write "Load parameters"(FALSE ("Load parameters")) -> ()
        n721 = Index Array(array="Saved AOD Raster Scan Parameter Sets", index=w1079) -> (element=w1078:T26)
        n722 = Unbundle By Name(w1078) -> ("Scan Range AOD (nm) 2"=w1077:dbl, "Step Size AOD (nm) 2"=w1076:dbl, "Scan Speed AOD (nm/s) 2"=w1075:dbl, "Number of scans (AOD) 2"=w1074:u16)
        n723 = flat-sequence {
          tunnel: w1077 -> [w1085]
          tunnel: w1076 -> [w1084]
          tunnel: w1075 -> [w1083]
          tunnel: w1074 -> [w1086]
          frame #0 {
            n724 = local write "Scan Speed (nm/s)"(w1083) -> ()
            n725 = local write "Scan Range (nm)"(w1085) -> ()
            n726 = local write "Step Size (nm)"(w1084) -> ()
          }
          frame #1 {
            n727 = property on="Number of F/B Scans (AOD)" class="DigNum (strict)"("Val(Sgnl)"=w1086) -> ()  [unwired: 2 in, 2 out]
          }
        }
      }
      event "Trap 1 (ON/OFF)", "Trap 2 (ON/OFF)": Value Change {
        n728 = event-data() -> ()  [unwired: 7 out]
        n729 = property on="Trap 2 ON" class="Bool (strict)"("Val(Sgnl)"="Trap 2 (ON/OFF)") -> ()  [unwired: 2 in, 2 out]
        n730 = property on="Trap 1 ON" class="Bool (strict)"("Val(Sgnl)"="Trap 1 (ON/OFF)") -> ()  [unwired: 2 in, 2 out]
      }
      event "DIO count 1 (ticks)", "DIO count 2 (ticks)", "DIO count 3 (ticks)", "Interlace", "Number Interlace Sets", "Not-Interlacing Set": Value Change {
        n731 = event-data() -> ()  [unwired: 7 out]
        n732 = local read "DIO count 3 (ticks)"() -> (w1099:u32)
        n733 = local read "DIO count 1 (ticks)"() -> (w1101:u32)
        n734 = local read "DIO count 2 (ticks)"() -> (w1100:u32)
        n735 = To Unsigned Byte Integer(number="Not-Interlacing Set") -> (unsigned 8bit integer=w1090:u8)
        n736 = Add(x=w1090, y=u8 1) -> (x+y=w1094:u8)
        n737 = xnode "Read/Write Control"("FPGA VI Reference In"=w1105, "error in"=w1103, "DIO count 1 (ticks)"=w1101, "DIO count 2 (ticks)"=w1100, "DIO count 3 (ticks)"=w1099, "Interlace ON/OFF"="Interlace", "Number Interlace Cycles"="Number Interlace Sets", "Interlace Off Parameters"=w1094) -> ("error out"=w1104:errorcluster)  [unwired: 1 out]
        n738 = Build Array(w1101, w1100, w1099) -> (w1092:u32[])
        n739 = Split 1D Array(array=w1092, index="Number Interlace Sets") -> (first subarray=w1102:u32[])  [unwired: 1 out]
        n740 = Index Array(array=w1092, index=w1090) -> (element=w1091:u32)
        n741 = Add Array Elements(numeric array=w1102) -> (sum=w1096:u32)
        n742 = Select(t=w1096, s="Interlace", f=w1091) -> (s? t:f=→"Total Counts (ticks)":u32)
      }
      event "Reset Feedback": Value Change {
        n743 = event-data() -> ()  [unwired: 7 out]
        n744 = Unbundle By Name("Reset Feedback") -> ("Set 1"=w1109:bool, "Set 2"=w1108:bool)
        n745 = xnode "Read/Write Control"("FPGA VI Reference In"=w1111, "error in"=w1106, "FB Reset Set 1"=w1109, "FB Reset Set 2"=w1108) -> ("error out"=w1107:errorcluster)  [unwired: 1 out]
      }
      event "PID Gains": Value Change {
        n746 = event-data() -> ()  [unwired: 7 out]
        n747 = Unbundle By Name("PID Gains") -> ("Set 1"=w1115:T14, "Set 2"=w1114:T14)
        n748 = xnode "Read/Write Control"("FPGA VI Reference In"=w1116, "error in"=w1112, "FB Gains Set 1"=w1115, "FB Gains Set 2"=w1114) -> ("error out"=w1113:errorcluster)  [unwired: 1 out]
      }
      event "AI2 to Setpoint", "Setpoints (V)": Value Change {
        n749 = event-data() -> ()  [unwired: 7 out]
        n750 = xnode "Read/Write Control"("FPGA VI Reference In"=w1122, "error in"=w1118) -> ("FPGA VI Reference Out"=w1121:T19, "error out"=w1120:errorcluster, "AI2 Y Sum Set 1"=w1129:i16, "AI2 Y Sum Set 2"=w1128:i16)
        n751 = Cluster To Array(cluster="AI2 to Setpoint") -> (array=w1132:bool[])
        n752 = local read "AI2 (V)"() -> (w1130:cluster{"Set 1":dbl, "Set 2":dbl})
        n753 = Or Array Elements(Boolean array=w1132) -> (logical OR=w1133:bool)
        n754 = Bundle By Name(cluster=w1130, "Set 1"=w1129, "Set 2"=w1128) -> (w1127:cluster{"Set 1":dbl, "Set 2":dbl})
        n755 = Divide(x=w1127, y=3276.7) -> (x/y=w1126:cluster{"Set 1":dbl, "Set 2":dbl})
        "AI2 (V)" <- w1126
        n756 = case shown="True" w1133 {
          tunnel: [w1136 w1153] -> w1125
          tunnel: "AI2 to Setpoint" -> [_ w1149]
          tunnel: "Setpoints (V)" -> [w1137 w1152]
          tunnel: w1126 -> [_ w1146]
          frame False {
            n757 = Multiply(x=3276.7, y=w1137) -> (x*y=w1138:cluster{"Set 1":dbl, "Set 2":dbl})
            n758 = To Word Integer(number=w1138) -> (16bit integer=w1136:cluster{"Set 1":i16, "Set 2":i16})
          }
          frame True {
            n759 = Unbundle By Name(w1146) -> ("Set 1"=w1145:dbl, "Set 2"=w1144:dbl)
            n760 = Unbundle By Name(w1152) -> ("Set 1"=w1151:dbl, "Set 2"=w1150:dbl)
            n761 = Unbundle By Name(w1149) -> ("Set 1"=w1148:bool, "Set 2"=w1147:bool)
            n762 = Select(t=w1145, s=w1148, f=w1151) -> (s? t:f=w1143:dbl)
            n763 = Select(t=w1144, s=w1147, f=w1150) -> (s? t:f=w1142:dbl)
            n764 = Bundle By Name(cluster=w1152, "Set 1"=w1143, "Set 2"=w1142) -> (w1140:cluster{"Set 1":dbl, "Set 2":dbl})
            n765 = local write "Setpoints (V)"(w1140) -> ()
            n766 = Multiply(x=3276.7, y=w1140) -> (x*y=w1141:cluster{"Set 1":dbl, "Set 2":dbl})
            n767 = To Word Integer(number=w1141) -> (16bit integer=w1153:cluster{"Set 1":i16, "Set 2":i16})
          }
        }
        n768 = Unbundle By Name(w1125) -> ("Set 1"=w1124:i16, "Set 2"=w1123:i16)
        n769 = xnode "Read/Write Control"("FPGA VI Reference In"=w1121, "error in"=w1120, "FB Setpoint Set 1"=w1124, "FB Setpoint Set 2"=w1123) -> ("error out"=w1119:errorcluster)  [unwired: 1 out]
      }
      event "Invert GI": Value Change {
        n770 = event-data() -> ()  [unwired: 7 out]
        n771 = xnode "Read/Write Control"("FPGA VI Reference In"=w1158, "error in"=w1156, "Invert GI"="Invert GI", "Invert GI 2"="Invert GI") -> ("error out"=w1157:errorcluster)  [unwired: 1 out]
      }
      event "Green FB Setpoint (mV)", "Green FB Gains", "Green FB On/Off", "Current When FB OFF (%)", "Green int current ON count adj": Value Change {
        n772 = event-data() -> ()  [unwired: 7 out]
        n773 = local read "Green FB Setpoint (mV)"() -> (w1165:dbl)
        n774 = local read "Current When FB OFF (%)"() -> (w1168:dbl)
        n775 = Multiply(x=w1165, y=3.2767) -> (x*y=w1164:dbl)
        n776 = Multiply(x=w1168, y=655.35) -> (x*y=w1169:dbl)
        n777 = To Unsigned Word Integer(number=w1169) -> (unsigned 16bit integer=w1167:u16)
        n778 = local read "Green int current ON count adj"() -> (w1172:u32)
        n779 = local read "Green FB Gains"() -> (w1171:T14)
        n780 = local read "Green Laser ON/Interlacing"() -> (w1162:bool)
        n781 = local read "Green laser mode"() -> (w1161:enum32{"Laser ON", "Laser OFF", "Interlace"})
        n782 = local read "Green FB On/Off"() -> (w1173:bool)
        n783 = Equal?(x=w1161, y=enum32{"Laser ON", "Laser OFF", "Interlace"}."Interlace") -> (x = y?=w1159:bool)
        n784 = Compound Arithmetic op=AND(w1159, w1173, w1162) -> (w1163:bool)
        n785 = xnode "Read/Write Control"("FPGA VI Reference In"=w1176, "error in"=w1175, "Green FB Setpoint"=w1164, "Green FB On/Off"=w1163, "Current Out"=w1167, "Green int current ON count adj"=w1172, "Green FB Gains"=w1171) -> ("error out"=w1174:errorcluster)  [unwired: 1 out]
      }
      event "Green laser mode", "Green Laser ON/Interlacing": Value Change {
        n786 = event-data() -> ()  [unwired: 7 out]
        n787 = case shown="True" "Green Laser ON/Interlacing" {
          tunnel: "Green laser mode" -> [_ w1190]
          tunnel: [enum32{"Laser ON", "Laser OFF", "Interlace"}."Laser OFF" ("Green laser mode") w1190] -> w1178
          tunnel: [FALSE w1186] -> w1177
          frame False {
          }
          frame True {
            n788 = local read "Green FB On/Off"() -> (w1187:bool)
            n789 = Equal?(x=w1190, y=enum32{"Laser ON", "Laser OFF", "Interlace"}."Interlace") -> (x = y?=w1188:bool)
            n790 = And(x=w1188, y=w1187) -> (x .and. y?=w1186:bool)
          }
        }
        n791 = xnode "Read/Write Control"("FPGA VI Reference In"=w1183, "error in"=w1181, "Operating Mode"=w1178, "Operating Mode 2"=w1178, "Green FB On/Off"=w1177) -> ("error out"=w1182:errorcluster)  [unwired: 1 out]
      }
      event "Test ttrig": Value Change {
        n792 = event-data() -> ()  [unwired: 7 out]
        n793 = xnode "Read/Write Control"("FPGA VI Reference In"=w1194, "error in"=w1193, "TTrig?"=TRUE) -> ("error out"=w1192:errorcluster)  [unwired: 1 out]
      }
      event "Neg. TTrig FPGA": Value Change {
        n794 = event-data() -> ()  [unwired: 7 out]
        n795 = xnode "Read/Write Control"("FPGA VI Reference In"=w1198, "error in"=w1197, "TTrig Negate Pos"="Neg. TTrig FPGA") -> ()  [unwired: 2 out]
      }
      event "- phase (APD 1 Gate)", "+ phase (APD 1 Gate)": Value Change {
        n796 = event-data() -> ()  [unwired: 7 out]
        n797 = local read "Phase Adj. (APD 1 Gate)"() -> (w1199:i16)
        n798 = Negate(x=w1199) -> (-x=w1207:i16)
        n799 = Select(t=w1207, s="- phase (APD 1 Gate)", f=w1199) -> (s? t:f=w1206:i16)
        n800 = Or(x="- phase (APD 1 Gate)", y="+ phase (APD 1 Gate)") -> (x .or. y?=w1202:bool)
        n801 = xnode "Read/Write Control"("FPGA VI Reference In"=w1209, "error in"=w1208, "Phase count adjustment (APD 1 Gate)"=w1206) -> ("FPGA VI Reference Out"=w1204:T19, "error out"=w1205:errorcluster)
        n802 = xnode "Read/Write Control"("FPGA VI Reference In"=w1204, "error in"=w1205, "+ phase (APD 1 Gate)"=w1202) -> ("error out"=w1203:errorcluster)  [unwired: 1 out]
      }
      event "+ phase (APD 2 Gate)", "- phase (APD 2 Gate)": Value Change {
        n803 = event-data() -> ()  [unwired: 7 out]
        n804 = local read "Phase Adj. (APD 2 Gate)"() -> (w1210:i16)
        n805 = Negate(x=w1210) -> (-x=w1218:i16)
        n806 = Select(t=w1218, s="- phase (APD 2 Gate)", f=w1210) -> (s? t:f=w1217:i16)
        n807 = Or(x="- phase (APD 2 Gate)", y="+ phase (APD 2 Gate)") -> (x .or. y?=w1213:bool)
        n808 = xnode "Read/Write Control"("FPGA VI Reference In"=w1220, "error in"=w1219, "Phase count adjustment (APD 2 Gate)"=w1217) -> ("FPGA VI Reference Out"=w1215:T19, "error out"=w1216:errorcluster)
        n809 = xnode "Read/Write Control"("FPGA VI Reference In"=w1215, "error in"=w1216, "+ phase (APD 2 Gate)"=w1213) -> ("error out"=w1214:errorcluster)  [unwired: 1 out]
      }
      event "Phase Adj. (APD Acq)", "+ phase (APD Acq)", "- phase (APD Acq)": Value Change {
        n810 = event-data() -> ()  [unwired: 7 out]
        n811 = local read "Phase Adj. (APD Acq)"() -> (w1223:i16)
        n812 = Negate(x=w1223) -> (-x=w1229:i16)
        n813 = Select(t=w1229, s="+ phase (APD Acq)", f=w1223) -> (s? t:f=w1228:i16)
        n814 = Or(x="+ phase (APD Acq)", y="- phase (APD Acq)") -> (x .or. y?=w1224:bool)
        n815 = xnode "Read/Write Control"("FPGA VI Reference In"=w1231, "error in"=w1230, "Phase Count Adjustment (APD Acq)"=w1228) -> ("FPGA VI Reference Out"=w1226:T19, "error out"=w1227:errorcluster)
        n816 = xnode "Read/Write Control"("FPGA VI Reference In"=w1226, "error in"=w1227, "+ phase (APD Acq)"=w1224) -> ("error out"=w1225:errorcluster)  [unwired: 1 out]
      }
      event "Phase adj. (GI)", "+ phase (GI)", "- phase (GI)": Value Change {
        n817 = event-data() -> ()  [unwired: 7 out]
        n818 = Negate(x="Phase adj. (GI)") -> (-x=w1240:i16)
